vi "fan_vi.vi"() -> ()   [LabVIEW 2020]
panel:
  in  "Speed":u32(knob) scale=0.0..5.0
  in  "stop":bool
  out "Pict Ring":u16(ring)
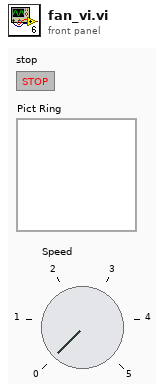
[diagram p1: front panel]
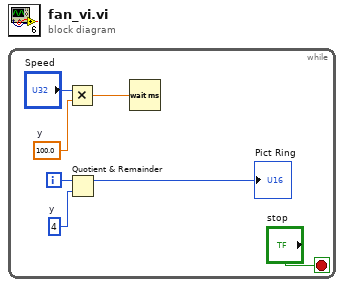
[diagram p0: block diagram]
diagram:
  n1 = while {
    i -> [w7]
    stop <- "stop" stop-if-true
    w2 = 100.0  # y
    w6 = 4  # y
    n2 = Multiply(x="Speed", y=w2) -> (x*y=w3:dbl)
    n3 = Quotient & Remainder(x=w7, y=w6) -> (x-y*floor(x/y)=→"Pict Ring":i32)  [unwired: 1 out]
    n4 = Wait (ms)(milliseconds to wait=w3) -> ()  [unwired: 1 out]
  }
